vi "MeasCfg.vi"(0 "DigitsIn":i32=5 caption="No of Digits" min=3 max=6 step=1, 1 "TauIn":dbl=5.0 caption="Tau / s" min=0.1 max=30.0 step=0.1 format="%.1f", 2 "PM16":bool, 3 "AvgIn":i32=100 caption="Averaging" min=1 max=100 step=1, 4 "TrigIn":dbl=5.0 caption="Trigger Level" min=1.0 max=100.0 format="%_3f", 5 "DiaIn":dbl=5.0 caption="D" min=0.0 format="%_4f", 6 "AttIn":dbl caption="Attenuation" min=-60.0 max=60.0 step=1.0 format="%#.3f", 7 "Type":u16, 8 "VISA In":refnum<visa-resource-name>, 9 "Sensor?":bool, 10 "Adapter":enum32{"PD", "TH", "PY"}(radio), 11 "BWIn":u16(ring) caption="Bandwidth" items=["HIGH", "LOW"], 13 "Tau?":bool, 14 "ACCIn":string(combo)="AUTO" caption="Accelerator") -> (12 "Ini":bool, 15 "DiaSet":dbl, 16 "ACCOut":string, 17 "BWOut":u16(ring) items=["HIGH", "LOW"], 19 "AttOut":dbl caption="Attenuation" format="%_4f", 20 "DigitsOut":i32, 21 "AvgOut":i32=100, 23 "TauIOut":dbl=5.0 caption="Tau" format="%_4f", 24 "TrigOut":dbl=5.0 caption="Trig", 25 "DiaOut":dbl=5.0 caption="Beam Dia", 27 "AOutcm²":dbl=5.0)   [LabVIEW 2011]
panel:
  out "AdapterOut":enum32{"PD", "TH", "PY"}(radio)
  out "Zero":dbl format="%#_4p"
  in  "DiaIn 2":dbl=5.0 caption="Y" format="%_4f"
  in  "Beam Setup":T1(radio)
  in  "Zero":bool
  in  "stop":bool
  # "Configure Measurement"
  # "Pyro:\n- Trigger"
  # "General\n- Beam Dia\n- Zero Adj"
  # "Thermo:\n- Accelerator"
  # "Photo:\n- Bandwidth"
  # "- No of Digits\n- Averaging Rate"
  # "dB"
  # "mm"
  # "mm"
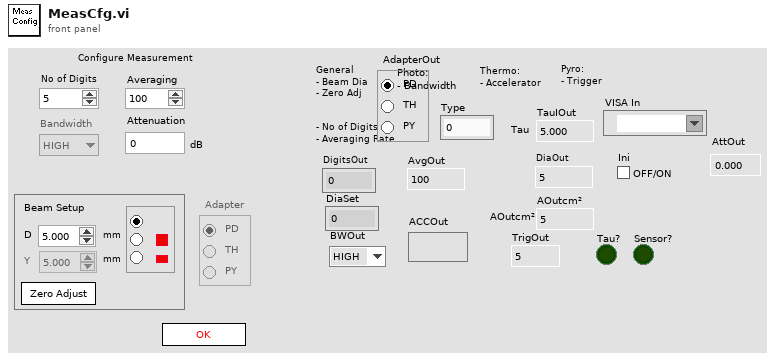
[diagram p1: front panel]
types:
  T1 = enum32{"Radio Selection 1", "Radio Selection 2", "Radio Selection 3"}
  T2 = enum8{"Enabled", "Disabled", "Disabled and Grayed Out"}
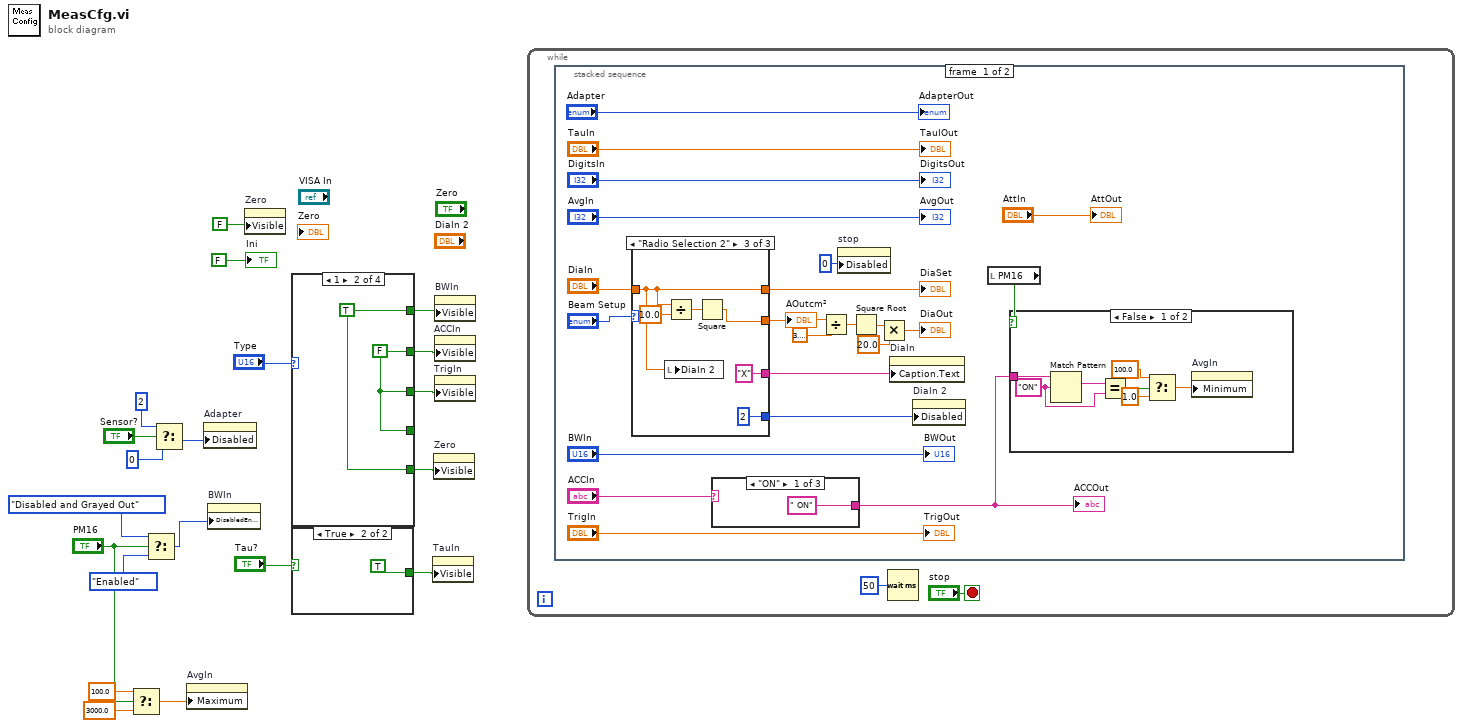
[diagram p0: block diagram]
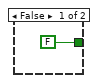
[diagram p2: hidden frame]
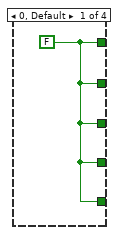
[diagram p3: hidden frame]
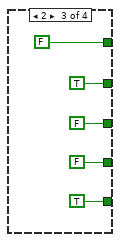
[diagram p4: hidden frame]
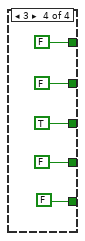
[diagram p5: hidden frame]
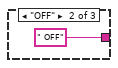
[diagram p7: hidden frame]
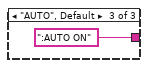
[diagram p8: hidden frame]
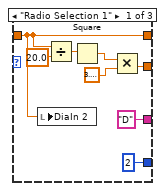
[diagram p9: hidden frame]
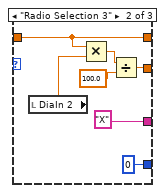
[diagram p10: hidden frame]
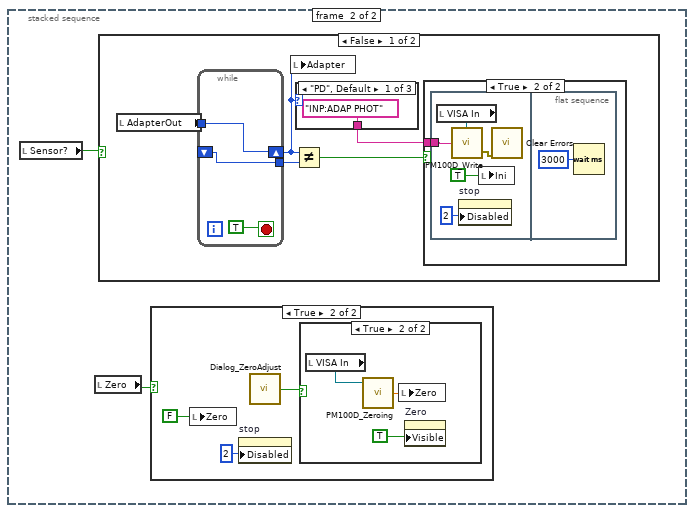
[diagram p11: hidden frame]
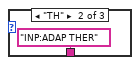
[diagram p12: hidden frame]
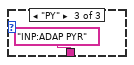
[diagram p13: hidden frame]
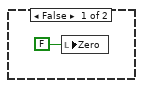
[diagram p16: hidden frame]
diagram:
  n1 = Select(t=100.0, s="PM16", f=3000.0) -> (s? t:f=w4:dbl)
  n2 = Select(t=T2."Disabled and Grayed Out", s="PM16", f=T2."Enabled" ("Disabled")) -> (s? t:f=w6:T2)
  n3 = Select(t=2, s="Sensor?", f=0) -> (s? t:f=w10:i32)
  n4 = property on="AvgIn" class="DigNum (strict)"("Maximum"=w4) -> ()  [unwired: 2 in, 2 out]
  n5 = property on="Adapter" class="RadioBtnsControl (strict)"("Disabled"=w10) -> ()  [unwired: 2 in, 2 out]
  n6 = property on="BWIn" class="Ring (strict)"("DisabledEnum"=w6) -> ()  [unwired: 2 in, 2 out]
  n7 = property on="Zero" class="DigNum (strict)"("Visible"=FALSE) -> ()  [unwired: 2 in, 2 out]
  n8 = case shown="1" "Type" {
    tunnel: [w21 w22 FALSE FALSE] -> w19
    tunnel: [w21 w23 TRUE FALSE] -> w18
    tunnel: [w21 w23 FALSE TRUE] -> w17
    tunnel: [w21 w23 FALSE FALSE] -> _
    tunnel: [w21 w22 TRUE FALSE] -> w16
    frame 0, Default {
      w21 = FALSE
    }
    frame 1 {
      w23 = FALSE
      w22 = TRUE
    }
    frame 2 {
    }
    frame 3 {
    }
  }
  n9 = case shown="True" "Tau?" {
    tunnel: [FALSE TRUE] -> w14
    frame False {
    }
    frame True {
    }
  }
  n10 = property on="TauIn" class="DigNum (strict)"("Visible"=w14) -> ()  [unwired: 2 in, 2 out]
  n11 = property on="Zero" class="Bool (strict)"("Visible"=w16) -> ()  [unwired: 2 in, 2 out]
  n12 = property on="BWIn" class="Ring (strict)"("Visible"=w19) -> ()  [unwired: 2 in, 2 out]
  n13 = property on="ACCIn" class="CmbBox"("Visible"=w18) -> ()  [unwired: 2 in, 2 out]
  n14 = property on="TrigIn" class="DigNum (strict)"("Visible"=w17) -> ()  [unwired: 2 in, 2 out]
  n15 = while {
    stop <- "stop" stop-if-true
    n16 = stacked-sequence {
      frame #0 {
        n17 = case shown="\"Radio Selection 2\"" "Beam Setup" {
          tunnel: [w71 w83 w86] -> w46
          tunnel: "DiaIn" -> [w71 w83 w86]
          tunnel: [w73 w81 w88] -> w53
          tunnel: ["D" "X" "X"] -> w56
          tunnel: [2 0 2] -> w55
          frame "Radio Selection 1" {
            n18 = local write "DiaIn 2"(w71) -> ()
            n19 = Divide(x=w71, y=20.0) -> (x/y=w76:dbl)
            n20 = Square(x=w76) -> (x^2=w75:dbl)
            n21 = Multiply(x=w75, y=3.141592653589793) -> (x*y=w73:dbl)
          }
          frame "Radio Selection 3" {
            n22 = local read "DiaIn 2"() -> (w79:dbl)
            n23 = Multiply(x=w83, y=w79) -> (x*y=w82:dbl)
            n24 = Divide(x=w82, y=100.0) -> (x/y=w81:dbl)
          }
          frame "Radio Selection 2" {
            n25 = local write "DiaIn 2"(w86) -> ()
            n26 = Divide(x=w86, y=10.0) -> (x/y=w89:dbl)
            n27 = Square(x=w89) -> (x^2=w88:dbl)
          }
        }
        "AOutcm²" <- w53
        "DiaSet" <- w46
        n28 = case shown="\"ON\"" "ACCIn" {
          tunnel: [" ON" ("ACCOut") " OFF" ("ACCOut") ":AUTO ON" ("ACCOut")] -> w39
          frame "ON" {
          }
          frame "OFF" {
          }
          frame "AUTO", Default {
          }
        }
        "ACCOut" <- w39
        n29 = Divide(x=w53, y=3.141592653589793) -> (x/y=w51:dbl)
        n30 = property on="stop" class="Bool"("Disabled"=u8 0) -> ()  [unwired: 2 in, 2 out]
        n31 = Square Root(x=w51) -> (sqrt(x)=w50:dbl)
        n32 = Multiply(x=w50, y=20.0) -> (x*y=→"DiaOut":dbl)
        n33 = property on="DiaIn" class="DigNum (strict)"("Caption.Text"=w56) -> ()  [unwired: 2 in, 2 out]
        n34 = property on="DiaIn 2" class="DigNum (strict)"("Disabled"=w55) -> ()  [unwired: 2 in, 2 out]
        n35 = local read "PM16"() -> (w38:bool)
        n36 = case shown="False" w38 {
          tunnel: w39 -> [w66 _]
          frame False {
            w65 = "ON" ("regular expression")
            n37 = Match Pattern(string=w66, regular expression=w65) -> (match substring=w64:string)  [unwired: 1 in, 3 out]
            n38 = Equal?(x=w64, y=w65) -> (x = y?=w63:bool)
            n39 = Select(t=100.0, s=w63, f=1.0) -> (s? t:f=w62:dbl)
            n40 = property on="AvgIn" class="DigNum (strict)"("Minimum"=w62) -> ()  [unwired: 2 in, 2 out]
          }
          frame True {
          }
        }
        "DigitsOut" <- "DigitsIn"
        "AvgOut" <- "AvgIn"
        "TrigOut" <- "TrigIn"
        "BWOut" <- "BWIn"
        "TauIOut" <- "TauIn"
        "AdapterOut" <- "Adapter"
        "AttOut" <- "AttIn"
      }
      frame #1 {
        n41 = local read "Sensor?"() -> (w91:bool)
        n42 = local read "Zero"() -> (w92:bool)
        n43 = case shown="False" w91 {
          frame False {
            n44 = local read "AdapterOut"() -> (w94:enum32{"PD", "TH", "PY"})
            n45 = while {
              shift-right: [w109] -> w93
              shift-left: _ -> [w108]
              tunnel: w94 -> [w109]
              tunnel: [w108] -> w97
              stop <- TRUE stop-if-true
            }
            n46 = local write "Adapter"(w93) -> ()
            n47 = Not Equal?(x=w93, y=w97) -> (x != y?=w96:bool)
            n48 = case shown="\"PD\", Default" w93 {
              tunnel: ["INP:ADAP PHOT" "INP:ADAP THER" "INP:ADAP PYR"] -> w95
              frame "PD", Default {
              }
              frame "TH" {
              }
              frame "PY" {
              }
            }
            n49 = case shown="True" w96 {
              tunnel: w95 -> [_ w101]
              frame False {
              }
              frame True {
                n50 = flat-sequence {
                  tunnel: w101 -> [w105]
                  frame #0 {
                    n51 = local read "VISA In"() -> (w106:refnum<visa-resource-name>)
                    n52 = call "PM100D_Write.vi"("Command"=w105, "VISA in"=w106) -> ("error out"=w102:errorcluster)  [unwired: 1 in, 1 out]
                    n53 = property on="stop" class="Bool"("Disabled"=u8 2) -> ()  [unwired: 2 in, 2 out]
                    n54 = local write "Ini"(TRUE ("Ini")) -> ()
                    n55 = call <vilib>:"Clear Errors.vi"("error in (no error)"=w102) -> ()  [unwired: 6 in, 1 out]
                  }
                  frame #1 {
                    n56 = Wait (ms)(milliseconds to wait=u32 3000) -> ()  [unwired: 1 out]
                  }
                }
              }
            }
          }
          frame True {
          }
        }
        n57 = case shown="True" w92 {
          frame False {
            n58 = local write "Zero"(FALSE ("Zero")) -> ()
          }
          frame True {
            n59 = local write "Zero"(FALSE ("Zero")) -> ()
            n60 = property on="stop" class="Bool"("Disabled"=u8 2) -> ()  [unwired: 2 in, 2 out]
            n61 = call "Dialog_ZeroAdjust.vi"() -> ("OK"=w112:bool)  [unwired: 7 in]
            n62 = case shown="True" w112 {
              frame False {
              }
              frame True {
                n63 = local read "VISA In"() -> (w117:refnum<visa-resource-name>)
                n64 = call "PM100D_Zeroing.vi"("VISA In"=w117) -> ("ZeroValue"=w116:dbl)  [unwired: 4 in]
                n65 = local write "Zero"(w116) -> ()
                n66 = property on="Zero" class="DigNum (strict)"("Visible"=TRUE) -> ()  [unwired: 2 in, 2 out]
              }
            }
          }
        }
      }
    }
    n67 = Wait (ms)(milliseconds to wait=u32 50) -> ()  [unwired: 1 out]
  }
  "Ini" <- FALSE ("Ini")
